vi "DAC Run.vi"(8 "error in":errorcluster, 11 "DAC TEG Temp in":refnum<class "DAC TEG Temp.lvclass">) -> (0 "error out":errorcluster, 3 "DAC TEG Temp out":refnum<class "DAC TEG Temp.lvclass">)   [LabVIEW 2019, in "DAC.lvlib" / "DAC TEG Temp.lvclass"]
uses:
  DAC TEG Temp.lvclass
  DAC.lvclass
  Results/Results Method.ctl
  Results/Results.lvlib
  Results/Heat Flow Results/Heat Flow Results.lvclass
  C:/Users/krio/Documents/LV_Projects/test-stand/App/DAC/DAC.lvclass
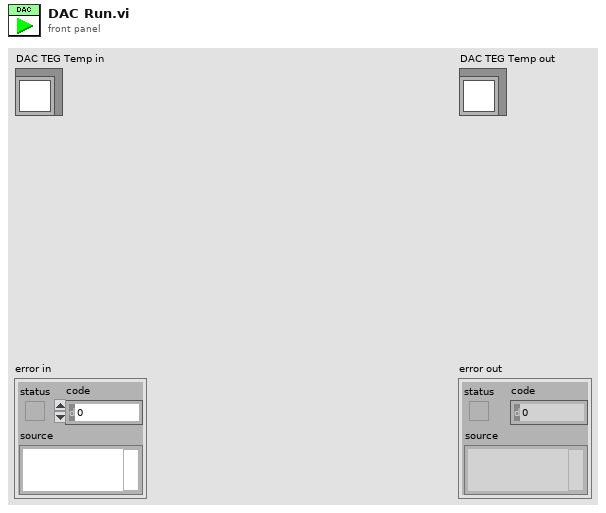
[diagram p1: front panel]
types:
  T1 = typedef "Results.lvlib/Results Method.ctl" = enum16{"Get", "Set"}
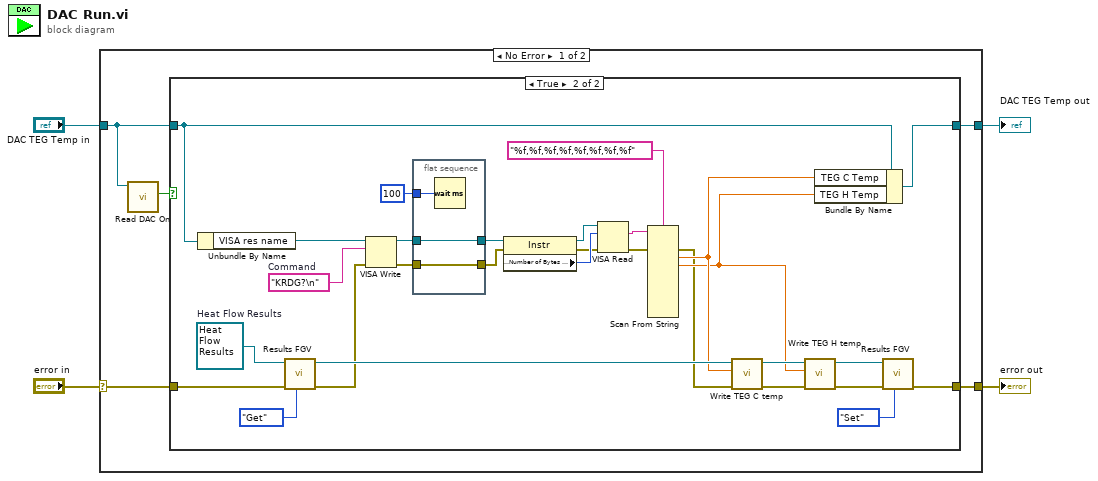
[diagram p0: block diagram]
diagram:
  n1 = case shown="No Error" "error in" {
    selector: "error in" -> [w7 w45]
    tunnel: [w6 w45] -> w2
    tunnel: [w8 w44] -> w1
    tunnel: "DAC TEG Temp in" -> [w5 w44]
    frame No Error {
      n2 = call "Read DAC On.vi"("DAC in"=w5) -> ("DAC On"=w9:bool)  [unwired: 8 in, 2 out]
      n3 = case shown="True" w9 {
        tunnel: w5 -> [w11 w39]
        tunnel: [w11 w40] -> w8
        tunnel: w7 -> [w10 w17]
        tunnel: [w10 w12] -> w6
        frame False {
        }
        frame True {
          w24 = refnum<class "Heat Flow Results.lvclass"> refnum  # Heat Flow Results
          w38 = "KRDG?\n"  # Command
          n4 = Unbundle By Name(w39) -> ("VISA res name"=w27:refnum<visa-resource-name>)
          n5 = call-dynamic "Results FGV.vi"("Method"=Results_Method."Get", "error in"=w17, "Results in"=w24) -> ("error out"=w16:errorcluster, "Results out"=w22:refnum<class "Heat Flow Results.lvclass">)  [unwired: 7 in]
          n6 = VISA Write(VISA resource name=w27, write buffer=w38, error in (no error)=w16) -> (VISA resource name out=w35:refnum<visa-resource-name>, error out=w36:errorcluster)  [unwired: 1 out]
          n7 = flat-sequence {
            tunnel: u32 100 ("milliseconds to wait") -> [w43]
            tunnel: w36 -> [w42]
            tunnel: [w42] -> w33
            tunnel: w35 -> [w41]
            tunnel: [w41] -> w34
            frame #0 {
              n8 = Wait (ms)(milliseconds to wait=w43) -> ()  [unwired: 1 out]
            }
          }
          n9 = property class="Instr"(reference=w34, error in=w33) -> (reference out=w32:refnum<visa-resource-name>, error out=w30:errorcluster, "Serial Settings:Number of Bytes at Serial Port"=w31:u32)
          n10 = VISA Read(VISA resource name=w32, byte count=w31, error in (no error)=w30) -> (read buffer=w29:string, error out=w26:errorcluster)  [unwired: 2 out]
          n11 = Scan From String(format string="%f,%f,%f,%f,%f,%f,%f,%f", input string=w29, error in=w26) -> (error out=w15:errorcluster, output 1=w19:dbl, output 2=w18:dbl)  [unwired: 15 in, 2 out]
          n12 = call "Write TEG C temp.vi"("error in (no error)"=w15, "TEG C temp"=w19, "Heat Flow Results in"=w22) -> ("error out"=w14:errorcluster, "Heat Flow Results out"=w21:refnum<class "Heat Flow Results.lvclass">)  [unwired: 7 in]
          n13 = call "Write TEG H temp.vi"("error in (no error)"=w14, "TEG H temp"=w18, "Heat Flow Results in"=w21) -> ("error out"=w13:errorcluster, "Heat Flow Results out"=w20:refnum<class "Heat Flow Results.lvclass">)  [unwired: 7 in]
          n14 = Bundle By Name(cluster=w39, "TEG C Temp"=w19, "TEG H Temp"=w18) -> (w40:refnum<class "DAC TEG Temp.lvclass">)
          n15 = call-dynamic "Results FGV.vi"("Method"=Results_Method."Set", "error in"=w13, "Results in"=w20) -> ("error out"=w12:errorcluster)  [unwired: 7 in, 1 out]
        }
      }
    }
    frame Error {
    }
  }
  "error out" <- w2
  "DAC TEG Temp out" <- w1
